vi "Z LQR_Subsystem.vi"(8 "State-Space Model":T1 {"Transport Delay" format="%.2f"; "D" format="%#.2g"; "C" format="%#.2g"; "B" format="%#.2g"; "A" format="%#.2g"; "properties"."Sampling Time" format="%#.6p"; "properties"."Output Delays" format="%.4f"; "properties"."Input Delays" format="%.4f"}, 9 "reset? alt":bool, 10 "Setpoint Alt":dbl[](array[numeric]), 11 "Stochastic State-Space Model":T3={"Sampling Time (s)"=1.0, "G"=[[1.0]], "B"=[[1.0]], "A"=[[0.9]], "C"=[[1.0]], "D"=[[0.0]], "H"=[[0.0]]}) -> (0 "Controller Action ut":dbl[](array[numeric]) format="%#.2g", 2 "Optimal Gain (K) Alt":dbl[][](array[numeric]) format="%.2f", 3 "Altitude":dbl[](array[numeric]), 4 "Waveform Chart Altitude":waveform(dbl)[](graph), 6 "Eigenvalues Alt":cdb[](array[numeric]) format="%.2f", 7 "Closed-Loop Step Response LQR Altitude":cluster{"time":dbl[], dbl[]}[](graph))   [LabVIEW 2011]
uses:
  <vilib>/Simulation/DiscreteLinear/Implementation/NILVSim Discrete Stochastic State Space.llb/NILVSim Discrete Stochastic State Space External Indirect Sim.vi
  <vilib>/Simulation/Implementation/XNodeFramework/SimXNode/SimX.xnode
  Control LQR.vi
  <vilib>/addons/Control Design/_Implementation/CD State Feedback Controller.vi
  <vilib>/addons/Control Design/_Implementation/NI_CD_Implementation.lvlib
  <vilib>/addons/Control Design/_Implementation/CD State Feedback Controller (Multiple Outputs).vi
  <vilib>/Simulation/SignalDisplay/Implementation/NILVSim Time Waveform.llb/SIM Time Waveform (vector).vi
  <vilib>/Simulation/Implementation/Shared/SIM Bundle Sim Info.vi
  <vilib>/Simulation/Implementation/Shared/SIM Unbundle Sim Info.vi
  <vilib>/Simulation/Implementation/Shared/NILVSim_Initialize.vi
  <vilib>/Simulation/Implementation/Shared/NILVSim_Manager.vi
  <vilib>/Simulation/Implementation/Shared/NI_SIM_Implementation.lvlib
  <vilib>/Simulation/Param Hierarchy/Typedefs/SIMPH Param Control Actions.ctl
  <vilib>/Simulation/Implementation/Shared/NILVSim_ParamChanged.vi
  <vilib>/Simulation/Implementation/Shared/SIM SimErrorHandler.vi
  <vilib>/Simulation/Implementation/Shared/NILVSim_FinalizeModel.vi
  <vilib>/Simulation/Implementation/Shared/NILVSim_GetModelError.vi
  <vilib>/Simulation/Implementation/Shared/SIMSCR Execution Mode.ctl
  <vilib>/Simulation/Scripting/Companion Diagram/SimConfigNode/SimDog.xnode
  <vilib>/Simulation/DiscreteLinear/Implementation/NILVSim Discrete Stochastic State Space.llb/SIM Discrete Stochastic State Space External Indirect Distributor Sim.vi
  <vilib>/Simulation/DiscreteLinear/Implementation/NILVSim Discrete Stochastic State Space.llb/SIM Discrete Stochastic State Space External Indirect Collector Sim.vi
  <vilib>/Simulation/Scripting/Companion Diagram/SimConfigNode/_simSolvers.ctl
  <vilib>/Simulation/Scripting/Companion Diagram/SimConfigNode/SimParams.ctl
  <vilib>/addons/Control Design/_Model Construction/Model Typedefs.llb/CD General Elements.ctl
  <vilib>/addons/Control Design/_Model Construction/NI_LinSys_Model Typedefs.lvlib
  <vilib>/addons/Control Design/_Model Construction/Model Typedefs.llb/CD State Space Model (MIMO).ctl
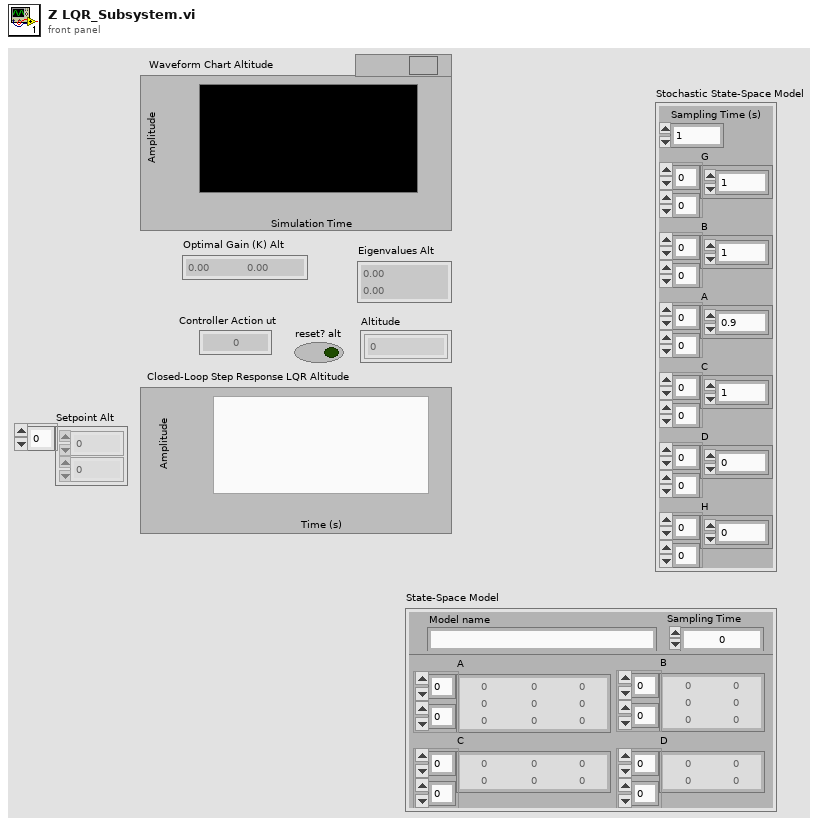
[diagram p1: front panel]
types:
  T1 = typedef "NI_LinSys_Model Typedefs.lvlib/CD State Space Model (MIMO).ctl" = cluster{"properties":T2, "A":dbl[][], "B":dbl[][], "C":dbl[][], "D":dbl[][], "StateNames":string[], "Transport Delay":dbl[][]}
  T2 = typedef "NI_LinSys_Model Typedefs.lvlib/CD General Elements.ctl" = cluster{"Model name":string, "Input names":string[], "Output names":string[], "Input Delays":dbl[], "Output Delays":dbl[], "Sampling Time":dbl, "Notes":string}
  T3 = cluster{"Sampling Time (s)":dbl, "G":dbl[][], "B":dbl[][], "A":dbl[][], "C":dbl[][], "D":dbl[][], "H":dbl[][]}
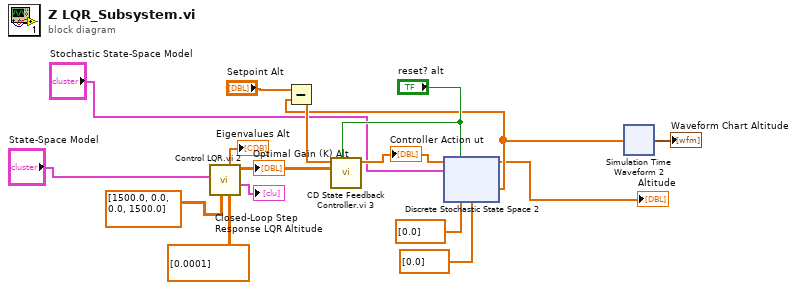
[diagram p0: block diagram]
diagram:
  n1 = call "Control LQR.vi 2"("R"=dbl[][] [[0.0001]], "Q"=dbl[][] [[1500.0, 0.0], [0.0, 1500.0]], "State-Space Model"="State-Space Model") -> ("Closed-Loop Step Response LQR"=→"Closed-Loop Step Response LQR Altitude":cluster{"time":dbl[], dbl[]}[], "Optimal Gain (K)"=w13:dbl[][], "Eigenvalues"=→"Eigenvalues Alt":cdb[])  [unwired: 5 in, 1 out]
  "Optimal Gain (K) Alt" <- w13
  n2 = Subtract(x="Setpoint Alt", y=w2) -> (x-y=w7:dbl[])
  n3 = call-poly "CD State Feedback Controller.vi 3"("Initialize"="reset? alt", "Controller Gain"=w13, "States"=w7) -> ("Controller Action"=w12:dbl[])  [unwired: 7 in, 1 out]
  "Controller Action ut" <- w12
  n4 = xnode ("Discrete Stochastic State Space 2")("Input u(k)"=w12, "reset?"="reset? alt", "Stochastic State-Space Model"="Stochastic State-Space Model", "Process Noise w(k)"=dbl[] [0.0], "Measurement Noise v(k)"=dbl[] [0.0]) -> ("Output y(k)"=→"Altitude":dbl[], "State x(k)"=w2:dbl[])  [unwired: 4 in, 1 out]
  n5 = xnode ("Simulation Time Waveform 2")("Value"=w2) -> ("Waveform Chart"=→"Waveform Chart Altitude":waveform(dbl)[])  [unwired: 1 in]
